vi "Add Connection To Connection List.vi"(8 "error in":errorcluster, 10 "data value reference":refnum<data-value>, 11 "TCP Slave in":refnum<class "TCP Server.lvclass">) -> (0 "error out":errorcluster)   [LabVIEW 2021, in "WebSockets.lvlib" / "TCP Server.lvclass"]
uses:
  TCP Server.lvclass
  Connection.ctl
  TCP Server.lvclass/TCP Server.ctl
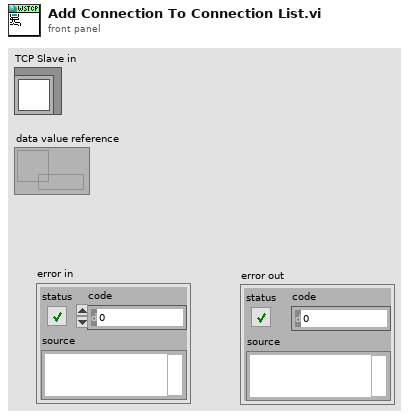
[diagram p1: front panel]
types:
  T1 = typedef "WebSockets.lvlib/TCP Server.lvclass/Connection Counter.ctl" = cluster{"Currently Connected":u32, "Connection Records":refnum<data-value>[]}
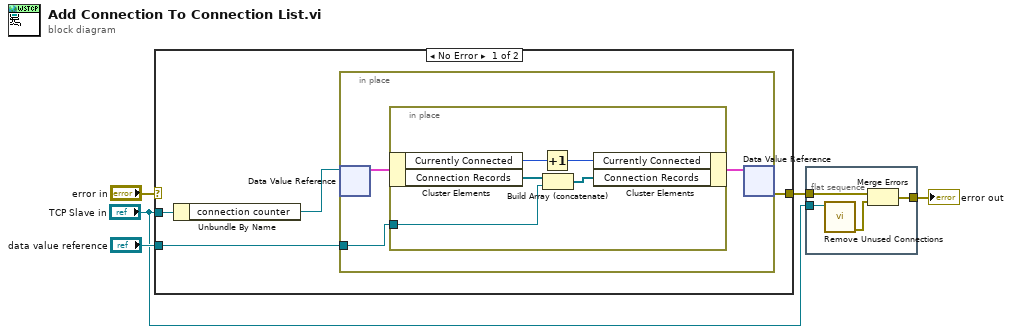
[diagram p0: block diagram]
diagram:
  n1 = case shown="No Error" "error in" {
    selector: "error in" -> [_ w18]
    tunnel: "data value reference" -> [w9 _]
    tunnel: [w7 w18] -> w2
    tunnel: "TCP Slave in" -> [w6 _]
    frame No Error {
      n2 = Unbundle By Name(w6) -> ("connection counter"=w8:refnum<data-value>)
      n3 = in-place {
        in-place-border: w9 -> [w10]
        n4 = in-place-dvr #1(w8) -> (w12:T1)  [unwired: 1 out]
        n5 = in-place {
          in-place-border: w10 -> [w13]
          n6 = in-place-cluster #2(w12) -> ("Currently Connected"=w17:u32, "Connection Records"=w15:refnum<data-value>[])
          n7 = Increment(x=w17) -> (x+1=w16:u32)
          n8 = Build Array (concatenate)(w15, w13) -> (w14:refnum<data-value>[])
          n9 = in-place-cluster #2("Currently Connected"=w16, "Connection Records"=w14) -> (w11:T1)
        }
        n10 = in-place-dvr #1(w11) -> (w7:errorcluster)  [unwired: 1 out]
      }
    }
    frame Error {
    }
  }
  n11 = flat-sequence {
    tunnel: [w22] -> w3
    tunnel: w2 -> [w21]
    tunnel: "TCP Slave in" -> [w19]
    frame #0 {
      n12 = call "Remove Unused Connections.vi"("TCP Slave in"=w19) -> ("error out"=w20:errorcluster)  [unwired: 10 in]
      n13 = Merge Errors(w21, w20) -> (w22:errorcluster)
    }
  }
  "error out" <- w3
